vi "Call DQMH Get Event Info VI.vi"(8 "error in":errorcluster, 11 "ProjectItem in":refnum<vi>) -> (0 "error out":errorcluster, 2 "Event Name":string, 4 "VI Ref":refnum<vi>)   [LabVIEW 2017, in "Open DQMH Request Message Diagram.lvlib"]
doc: "Calls get Event Info VI.\n\nBSD 3-Clause License\n\nCopyright (c) 2022, Neosoft Technologies Inc\nAll rights reserved.\n\nRedistribution and use in source and binary forms, with or without\nmodification, are permitted provided that the following conditions are met:\n\n1. Redistributions of source code must retain the above copyright notice, this\n list of conditions and the following disclaimer.\n\n2. Redistributions in binary form must reproduce the above copyright notice,\n this list of conditions and the following disclaimer in the documentation\n and/or other materials provided with the distribution.\n\n3. Neither the name of the copyright holder nor the names of its\n contributors may be used to endorse or promote products derived from\n this software without specific prior written permission.\n\nTHIS SOFTWARE IS PROVIDED BY THE COPYRIGHT HOLDERS AND CONTRIBUTORS \"AS IS\"\nAND ANY EXPRESS OR IMPLIED WARRANTIES, INCLUDING, BUT NOT LIMITED TO, THE\nIMPLIED WARRANTIES OF MERCHANTABILITY AND FITNESS FOR A PARTICULAR PURPOSE ARE\nDISCLAIMED. IN NO EVENT SHALL THE COPYRIGHT HOLDER OR CONTRIBUTORS BE LIABLE\nFOR ANY DIRECT, INDIRECT, INCIDENTAL, SPECIAL, EXEMPLARY, OR CONSEQUENTIAL\nDAMAGES (INCLUDING, BUT NOT LIMITED TO, PROCUREMENT OF SUBSTITUTE GOODS OR\nSERVICES; LOSS OF USE, DATA, OR PROFITS; OR BUSINESS INTERRUPTION) HOWEVER\nCAUSED AND ON ANY THEORY OF LIABILITY, WHETHER IN CONTRACT, STRICT LIABILITY,\nOR TORT (INCLUDING NEGLIGENCE OR OTHERWISE) ARISING IN ANY WAY OUT OF THE USE\nOF THIS SOFTWARE, EVEN IF ADVISED OF THE POSSIBILITY OF SUCH DAMAGE."
uses:
  Open DQMH Request Message Diagram.lvlib
  <vilib>/Utility/traverseref.llb/TRef TravTarget.ctl
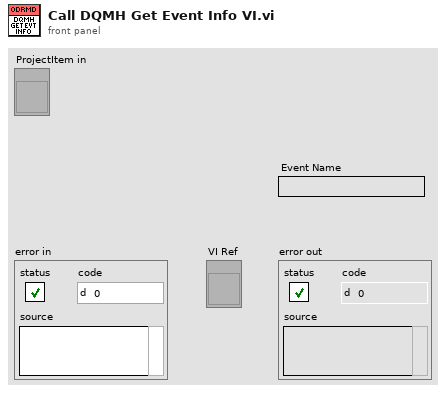
[diagram p1: front panel]
types:
  T1 = typedef "TRef TravTarget.ctl" = enum16{"FP", "BD", "Other"}
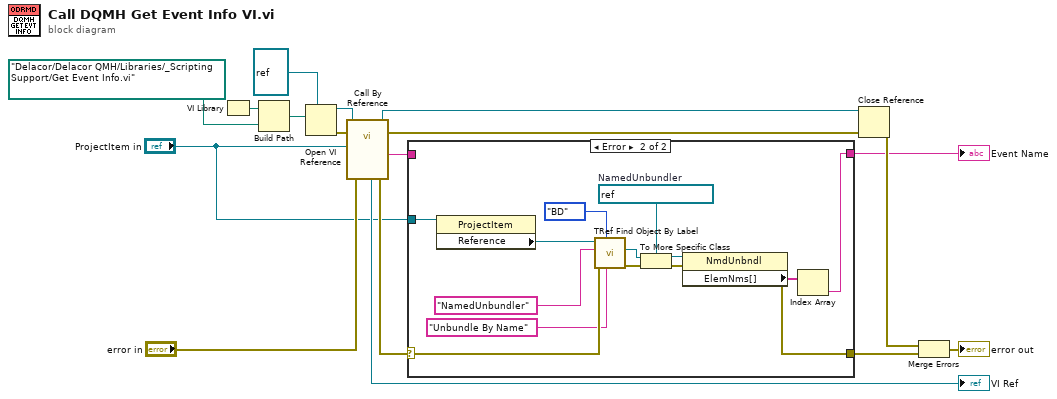
[diagram p0: block diagram]
diagram:
  n1 = VI Library() -> (path=w8:path)
  n2 = Build Path(base path=w8, name or relative path=path "Delacor/Delacor QMH/Libraries/_Scripting Support/Get Event Info.vi") -> (appended path=w7:path)
  n3 = Open VI Reference(type specifier VI Refnum (for type only)=refnum<vi> refnum, vi path=w7) -> (vi reference=w10:refnum<vi>, error out=w15:errorcluster)  [unwired: 4 in]
  n4 = call-by-ref "?"(reference=w10, error in=w15, 8:"error in (no error)"="error in", "ProjectItem in"="ProjectItem in") -> (reference out=w9:refnum<vi>, error out=w17:errorcluster, 0:"error out"=w12:errorcluster, "Event Name"=w4:string, "VI Ref"=→"VI Ref":refnum<vi>)  [unwired: 5 in, 2 out]
  n5 = case shown="Error" w12 {
    selector: w12 -> [w19 w30]
    tunnel: w4 -> [w18 _]
    tunnel: [w18 w21] -> w3
    tunnel: [w19 w31] -> w11
    tunnel: "ProjectItem in" -> [_ w20]
    frame No Error {
    }
    frame Error {
      w28 = refnum<vi> refnum  # NamedUnbundler
      n6 = property class="ProjectItem"(reference=w20) -> ("Reference"=w23:refnum<vi>)  [unwired: 1 in, 2 out]
      n7 = call <vilib>:"TRef Find Object By Label.vi"("Label"="Unbundle By Name" ("Class Name"), "Traverse Target"=TRef_TravTarget."BD", "error in (no error)"=w30, "Class Name"="NamedUnbundler", "VI Ref"=w23) -> ("error out"=w32:errorcluster, "Found Obj Ref"=w27:refnum<vi>)  [unwired: 3 in, 2 out]
      n8 = To More Specific Class(target class=w28, reference=w27, error in=w32) -> (specific class reference=w29:refnum<vi>, error out=w33:errorcluster)
      n9 = property class="NmdUnbndl"(reference=w29, error in=w33) -> (error out=w31:errorcluster, "ElemNms[]"=w24:string[])  [unwired: 1 out]
      n10 = Index Array(array=w24) -> (element=w21:string)  [unwired: 1 in]
    }
  }
  "Event Name" <- w3
  n11 = Close Reference(reference=w9, error in (no error)=w17) -> (error out=w16:errorcluster)
  n12 = Merge Errors(w16, w11) -> (→"error out":errorcluster)
